vi "WriteSamples.vi"(8 "error in (no error)":errorcluster, 10 "clSampleDataArray":T1, 11 "SaveWaveforms in":refnum<class "SaveWaveforms.lvclass">) -> (0 "error out":errorcluster, 3 "SaveWaveforms out":refnum<class "SaveWaveforms.lvclass">)   [LabVIEW 2014, in "AnalysisPlugins.lvlib" / "SaveWaveforms.lvclass"]
uses:
  SaveWaveforms.lvclass
  AnalysisPluginBaseClass/Typedefs/SampleDataInput.ctl
  AnalysisPluginBaseClass/AnalysisPluginsBase.lvclass
panel:
  out "Waveform Graph":waveform(dbl)[](graph)
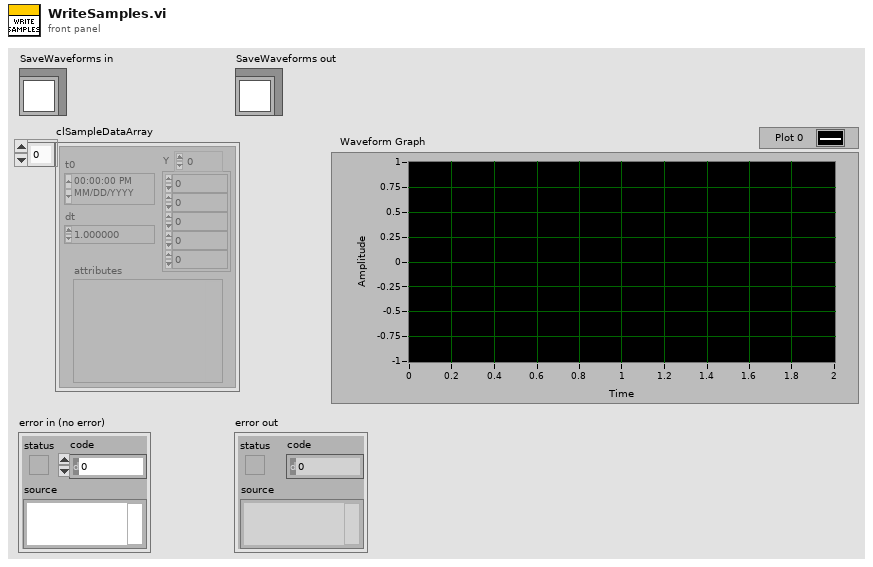
[diagram p1: front panel]
types:
  T1 = typedef "AnalysisPlugins.lvlib/AnalysisPluginsBase.lvclass/SampleDataInput.ctl" = waveform(dbl)[]
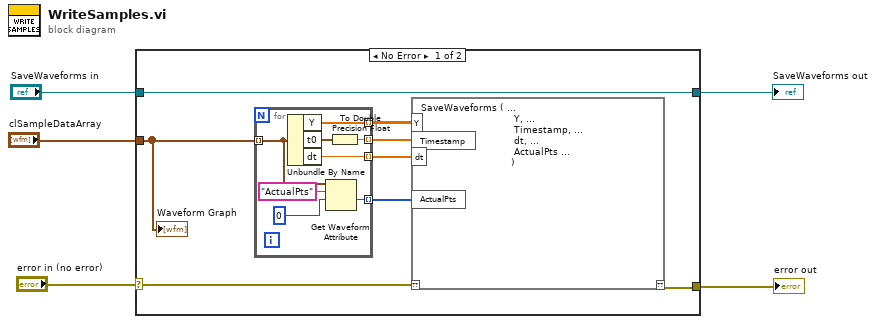
[diagram p0: block diagram]
diagram:
  n1 = case shown="No Error" "error in (no error)" {
    selector: "error in (no error)" -> [w7 w23]
    tunnel: [w6 w23] -> w4
    tunnel: [w12 w22] -> w2
    tunnel: "SaveWaveforms in" -> [w12 w22]
    tunnel: "clSampleDataArray" -> [w13 _]
    frame No Error {
      n2 = for {
        tunnel: w13 -> [w18] mode=indexing
        tunnel: [w21] -> w11 mode=indexing
        tunnel: [w14] -> w10 mode=indexing
        tunnel: [w19] -> w9 mode=indexing
        tunnel: [w15] -> w8 mode=indexing
        n3 = Unbundle By Name(w18) -> ("Y"=w21:dbl[], "t0"=w20:timestamp, "dt"=w19:dbl)
        n4 = Get Waveform Attribute(5:u32 0, 6:"ActualPts" ("name"), 7:w18) -> (1:w15:u32)  [unwired: 1 in, 3 out]
        n5 = To Double Precision Float(number=w20) -> (double precision float=w14:dbl)
      }
      n6 = script code="SaveWaveforms ( ...\n                               Y, ...\n                               Timestamp, ...\n                               dt, ...\n                               ActualPts ...\n                              )"("??"=w7, "Y"=w11, "Timestamp"=w10, "dt"=w9, "ActualPts"=w8) -> ("??"=w6:errorcluster)
      "Waveform Graph" <- w13
    }
    frame Error {
    }
  }
  "error out" <- w4
  "SaveWaveforms out" <- w2
